vi "Shoot Joystick.vi"(6 "Auto Calculate Speed":bool, 8 "High Speed":bool, 9 "Medium Speed":bool, 10 "Low Speed":bool, 11 "Raw Throttle":dbl) -> (3 "Shoot Teleop Command":T1)   [LabVIEW 2019]
uses:
  Shooter Command Type Def.ctl
  Shooter Mode Type Def.ctl
panel:
  in  "High":dbl
  in  "Medium":dbl
  in  "Low":dbl
  # "AUTO CALCULATE DOES NOT DO\nANYTHING RIGHT NOW"
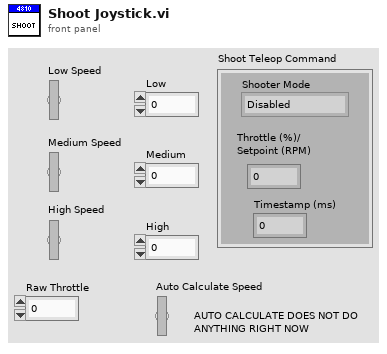
[diagram p1: front panel]
types:
  T1 = typedef "Shooter Command Type Def.ctl" = cluster{"Shooter Mode":T2, "Throttle (%)/ \nSetpoint (RPM)":dbl, "Timestamp (ms)":dbl}
  T2 = typedef "Shooter Mode Type Def.ctl" = enum16{"Disabled", "Raw Throttle", "Velocity Control"}
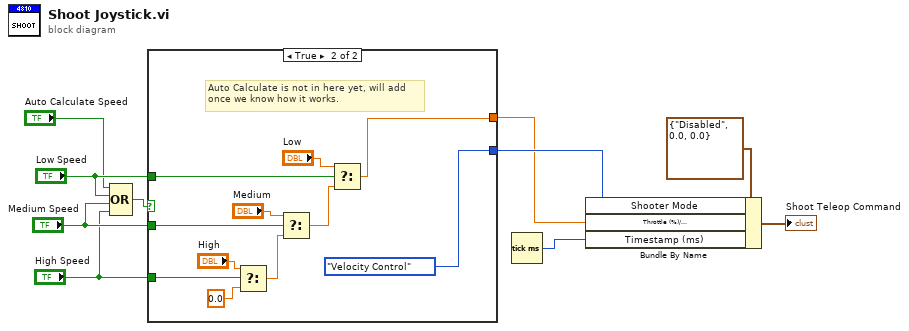
[diagram p0: block diagram]
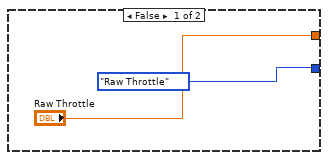
[diagram p2: hidden frame]
diagram:
  n1 = Compound Arithmetic op=OR("Auto Calculate Speed", "Low Speed", "Medium Speed", "High Speed") -> (w6:bool)
  n2 = case shown="True" w6 {
    tunnel: "High Speed" -> [_ w23]
    tunnel: "Medium Speed" -> [_ w22]
    tunnel: "Low Speed" -> [_ w21]
    tunnel: [Shooter_Mode_Type_Def."Raw Throttle" ("Shooter Mode") Shooter_Mode_Type_Def."Velocity Control" ("Shooter Mode")] -> w7
    tunnel: ["Raw Throttle" w13] -> w1
    frame False {
    }
    frame True {
      # "Auto Calculate is not in here yet, will add\nonce we know how it works."
      n3 = Select(t="High", s=w23, f=0.0) -> (s? t:f=w17:dbl)
      n4 = Select(t="Medium", s=w22, f=w17) -> (s? t:f=w16:dbl)
      n5 = Select(t="Low", s=w21, f=w16) -> (s? t:f=w13:dbl)
    }
  }
  n6 = Tick Count (ms)() -> (millisecond timer value=w8:u32)
  n7 = Bundle By Name(cluster=T1 {"Shooter Mode"=enum."Disabled", "Throttle (%)/ \nSetpoint (RPM)"=0.0, "Timestamp (ms)"=0.0} ("Teleop Shooter Command"), "Shooter Mode"=w7, "Throttle (%)/ \nSetpoint (RPM)"=w1, "Timestamp (ms)"=w8) -> (→"Shoot Teleop Command":T1)
